vi "Vision Research Phantom Series PhCon PhConfigCameraPool.vi"(0 "Period (ms)":u32=3000, 5 "Error In (no error)":errorcluster, 8 "Simulate? (False)":bool) -> (19 "Error Out":errorcluster)   [LabVIEW 2013, in "VRI.lvlib"]
doc: "Use this template to build a VI to interface with the PhCon dll. Configure the call library function for the desired function prototype.\n\nWritten by:\nBLOOMY CONTROLS, INC\nWINDSOR, CT 06095, USA\n860-298-9925\nwww.bloomy.com\nV1.0.0\nMay, 2004"
uses:
  VRI.lvlib
  Projects/SDK/32-bit/Vision Research Phantom Series Labview Driver/Phantom DLLs/PhCon.dll
panel:
  # "For instructions on the use of this VI, press Ctrl+H to display the help window and move the mouse over the icon, controls, and indicators"
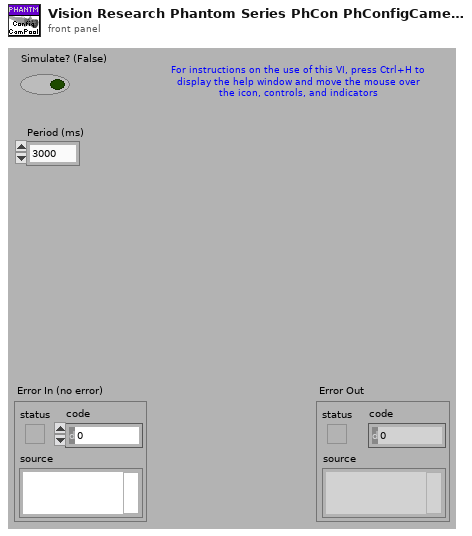
[diagram p1: front panel]
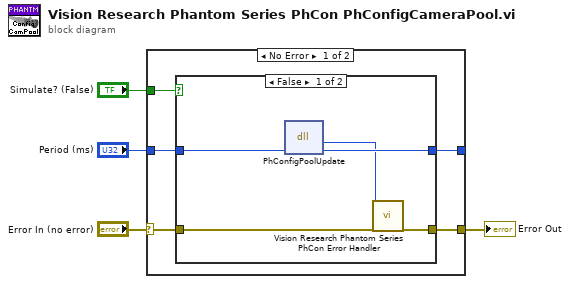
[diagram p0: block diagram]
diagram:
  n1 = case shown="No Error" "Error In (no error)" {
    selector: "Error In (no error)" -> [w9 w18]
    tunnel: [w8 w18] -> w3
    tunnel: "Simulate? (False)" -> [w7 _]
    tunnel: "Period (ms)" -> [w6 w17]
    tunnel: [w5 w17] -> _
    frame No Error {
      n2 = case shown="False" w7 {
        tunnel: w9 -> [w13 w16]
        tunnel: [w14 w16] -> w8
        tunnel: w6 -> [w12 w15]
        tunnel: [w11 w15] -> w5
        frame False {
          n3 = dll-call lib="C:/Projects/SDK/32-bit/Vision Research Phantom Series Labview Driver/Phantom DLLs/PhCon.dll" fn="PhConfigPoolUpdate"("Period"=w12) -> ("HRESULT"=w10:i32, "Period"=w11:u32)  [unwired: 3 in, 2 out]
          n4 = call "Vision Research Phantom Series PhCon Error Handler.vi"("ErrNo"=w10, "Error In (no error)"=w13) -> ("Error Out"=w14:errorcluster)  [unwired: 17 out]
        }
        frame True {
          # "It looks as though the dlls can provide simulated data so this case may not have to be used"
        }
      }
    }
    frame Error {
    }
  }
  "Error Out" <- w3
